vi "Launch SessionCore (Client).vi"(8 "error in (no error)":errorcluster, 11 "Session in":refnum<class "Session.lvclass">) -> (0 "error out":errorcluster, 2 "Session ID":i32, 3 "Session out":refnum<class "Session.lvclass">)   [LabVIEW 2013, in "MQTT Server.lvlib" / "Session.lvclass"]
uses:
  Session.lvclass
  process(Client).vi
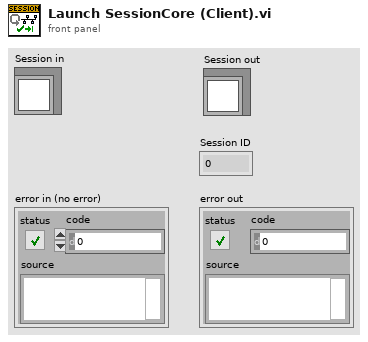
[diagram p1: front panel]
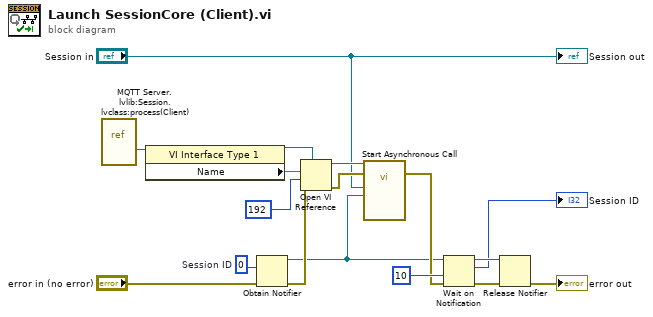
[diagram p0: block diagram]
diagram:
  w9 = 0  # Session ID
  n1 = vi-ref "MQTT Server.lvlib:Session.lvclass:process(Client).vi"() -> (w3:refnum<vi>)
  n2 = property class="VI Interface Type 1"(reference=w3) -> (reference out=w5:refnum<vi>, "Name"=w4:string)  [unwired: 1 in, 1 out]
  n3 = Obtain Notifier(notification data type=w9, error in (no error)="error in (no error)") -> (notifier out=w10:refnum<notifier>, error out=w15:errorcluster)  [unwired: 2 in, 1 out]
  n4 = Open VI Reference(type specifier VI Refnum (for type only)=w5, vi path=w4, options=192, error in (no error)=w15) -> (vi reference=w6:refnum<vi>, error out=w7:errorcluster)  [unwired: 2 in]
  n5 = call-by-ref "Start Asynchronous Call"(reference=w6, error in=w7, "Sync"=w10, "Session in"="Session in") -> (error out=w13:errorcluster)  [unwired: 8 in, 3 out]
  n6 = Wait on Notification(notifier=w10, timeout in ms (-1)=10, error in (no error)=w13) -> (notifier out=w11:refnum<notifier>, notification=→"Session ID":i32, error out=w14:errorcluster)  [unwired: 1 in, 1 out]
  n7 = Release Notifier(notifier=w11, error in (no error)=w14) -> (error out=→"error out":errorcluster)  [unwired: 1 in, 2 out]
  "Session out" <- "Session in"
